vi "t2.vi"() -> ()   [LabVIEW 2019]
uses:
  <vilib>/Utility/file.llb/Write Delimited Spreadsheet (I64).vi
panel:
  out "Array":i32[][](array[numeric])
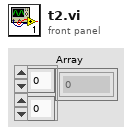
[diagram p1: front panel]
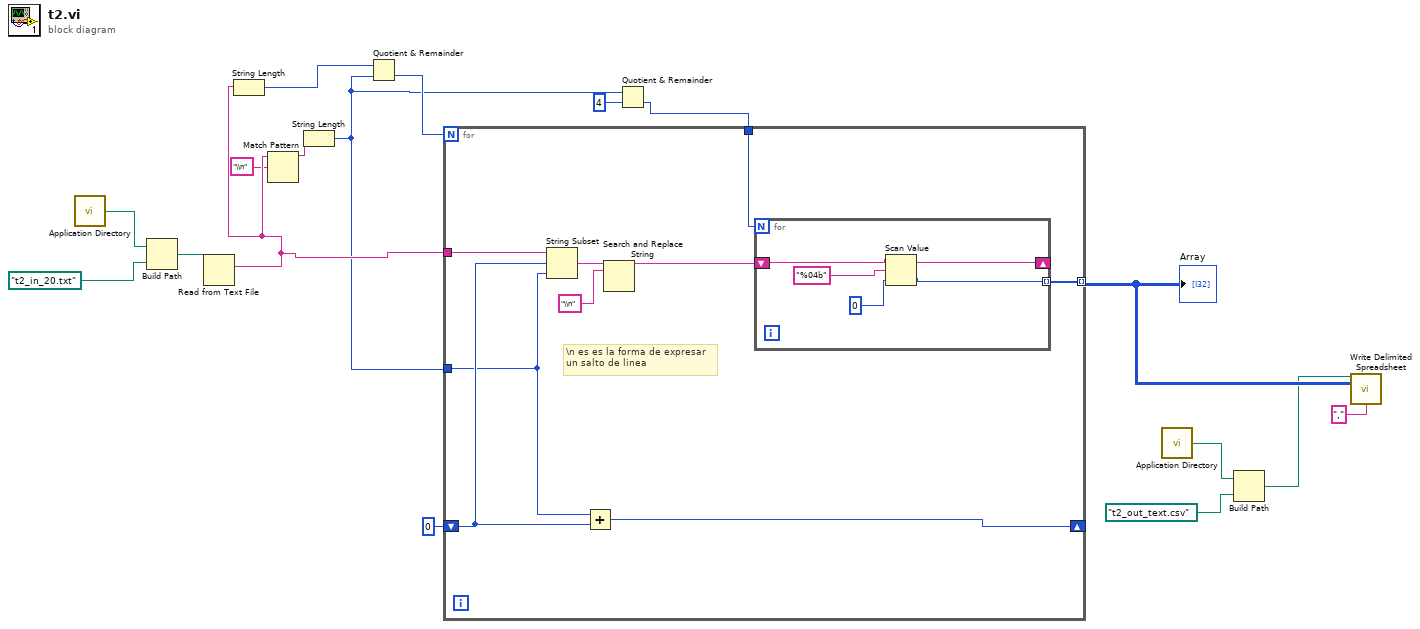
[diagram p0: block diagram]
diagram:
  n1 = call <vilib>:"Application Directory.vi"() -> ("Application Directory"=w17:path)
  n2 = Build Path(base path=w17, name or relative path=path "t2_in_20.txt" ("file (use dialog)")) -> (appended path=w15:path)
  n3 = Read from Text File(file (use dialog)=w15) -> (text=w8:string)  [unwired: 3 in, 3 out]
  n4 = String Length(string=w8) -> (length=w5:i32)
  n5 = Match Pattern(string=w8, regular expression="\\n") -> (before substring=w6:string)  [unwired: 1 in, 3 out]
  n6 = String Length(string=w6) -> (length=w1:i32)
  n7 = Quotient & Remainder(x=w5, y=w1) -> (floor(x/y)=w4:i32)  [unwired: 1 out]
  n8 = Quotient & Remainder(x=w1, y=4) -> (floor(x/y)=w2:i32)  [unwired: 1 out]
  n9 = for {
    N: w4 -> [_]
    tunnel: w8 -> [w26]
    shift-right: [w25] -> _
    shift-left: 0 -> [w24]
    tunnel: [w20] -> w13 mode=indexing
    tunnel: w2 -> [w19]
    tunnel: w1 -> [w18]
    # "\\n es es la forma de expresar\nun salto de linea"
    n10 = String Subset(string=w26, offset (0)=w24, length (rest)=w18) -> (substring=w23:string)
    n11 = Add(x=w18, y=w24) -> (x+y=w25:i32)
    n12 = Search and Replace String(input string=w23, search string="\\n" ("substring (\"\")")) -> (result string=w21:string)  [unwired: 6 in, 3 out]
    n13 = for {
      N: w19 -> [_]
      tunnel: [w28] -> w20 mode=indexing
      shift-right: [w30] -> _
      shift-left: w21 -> [w31]
      n14 = Scan Value(string=w31, format string="%04b", default (0 dbl)=0 ("length (rest)")) -> (output string=w30:string, value=w28:i32)
    }
  }
  "Array" <- w13
  n15 = call <vilib>:"Application Directory.vi"() -> ("Application Directory"=w12:path)
  n16 = Build Path(base path=w12, name or relative path=path "t2_out_text.csv" ("file (use dialog)")) -> (appended path=w10:path)
  n17 = call-poly <vilib>:"Write Delimited Spreadsheet.vi"("file path (dialog if empty)"=w10, "2D data"=w13, "delimiter (\\t)"="," ("delimiter (\\t)")) -> ()  [unwired: 11 in, 2 out]
